vi "Open file simple via system exec.vi"(0 "file path":path) -> (4 "command line":string, 15 "error out":errorcluster)   [LabVIEW 2013]
doc: "Opens the file via a simple System exec call.\nFails if hte file is already used by another process. Example: Access Database file is use by Prosis. Then this command fails."
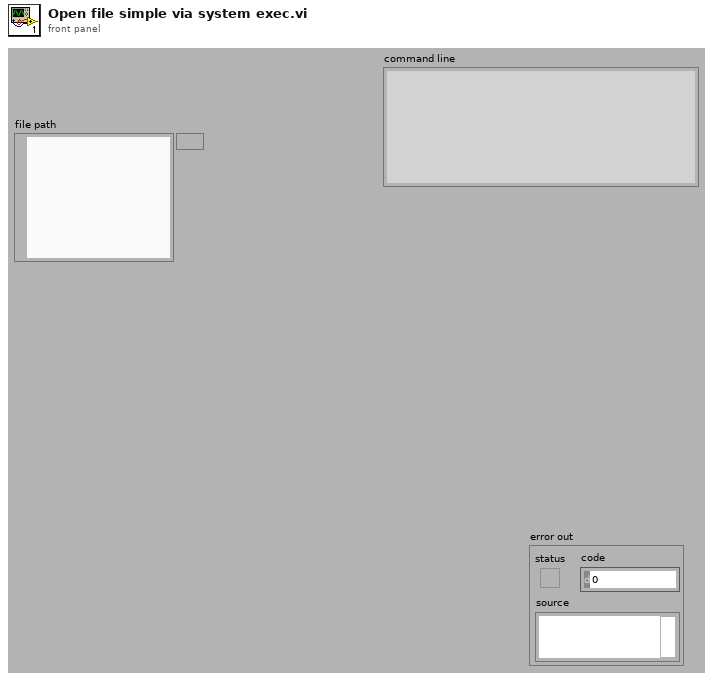
[diagram p1: front panel]
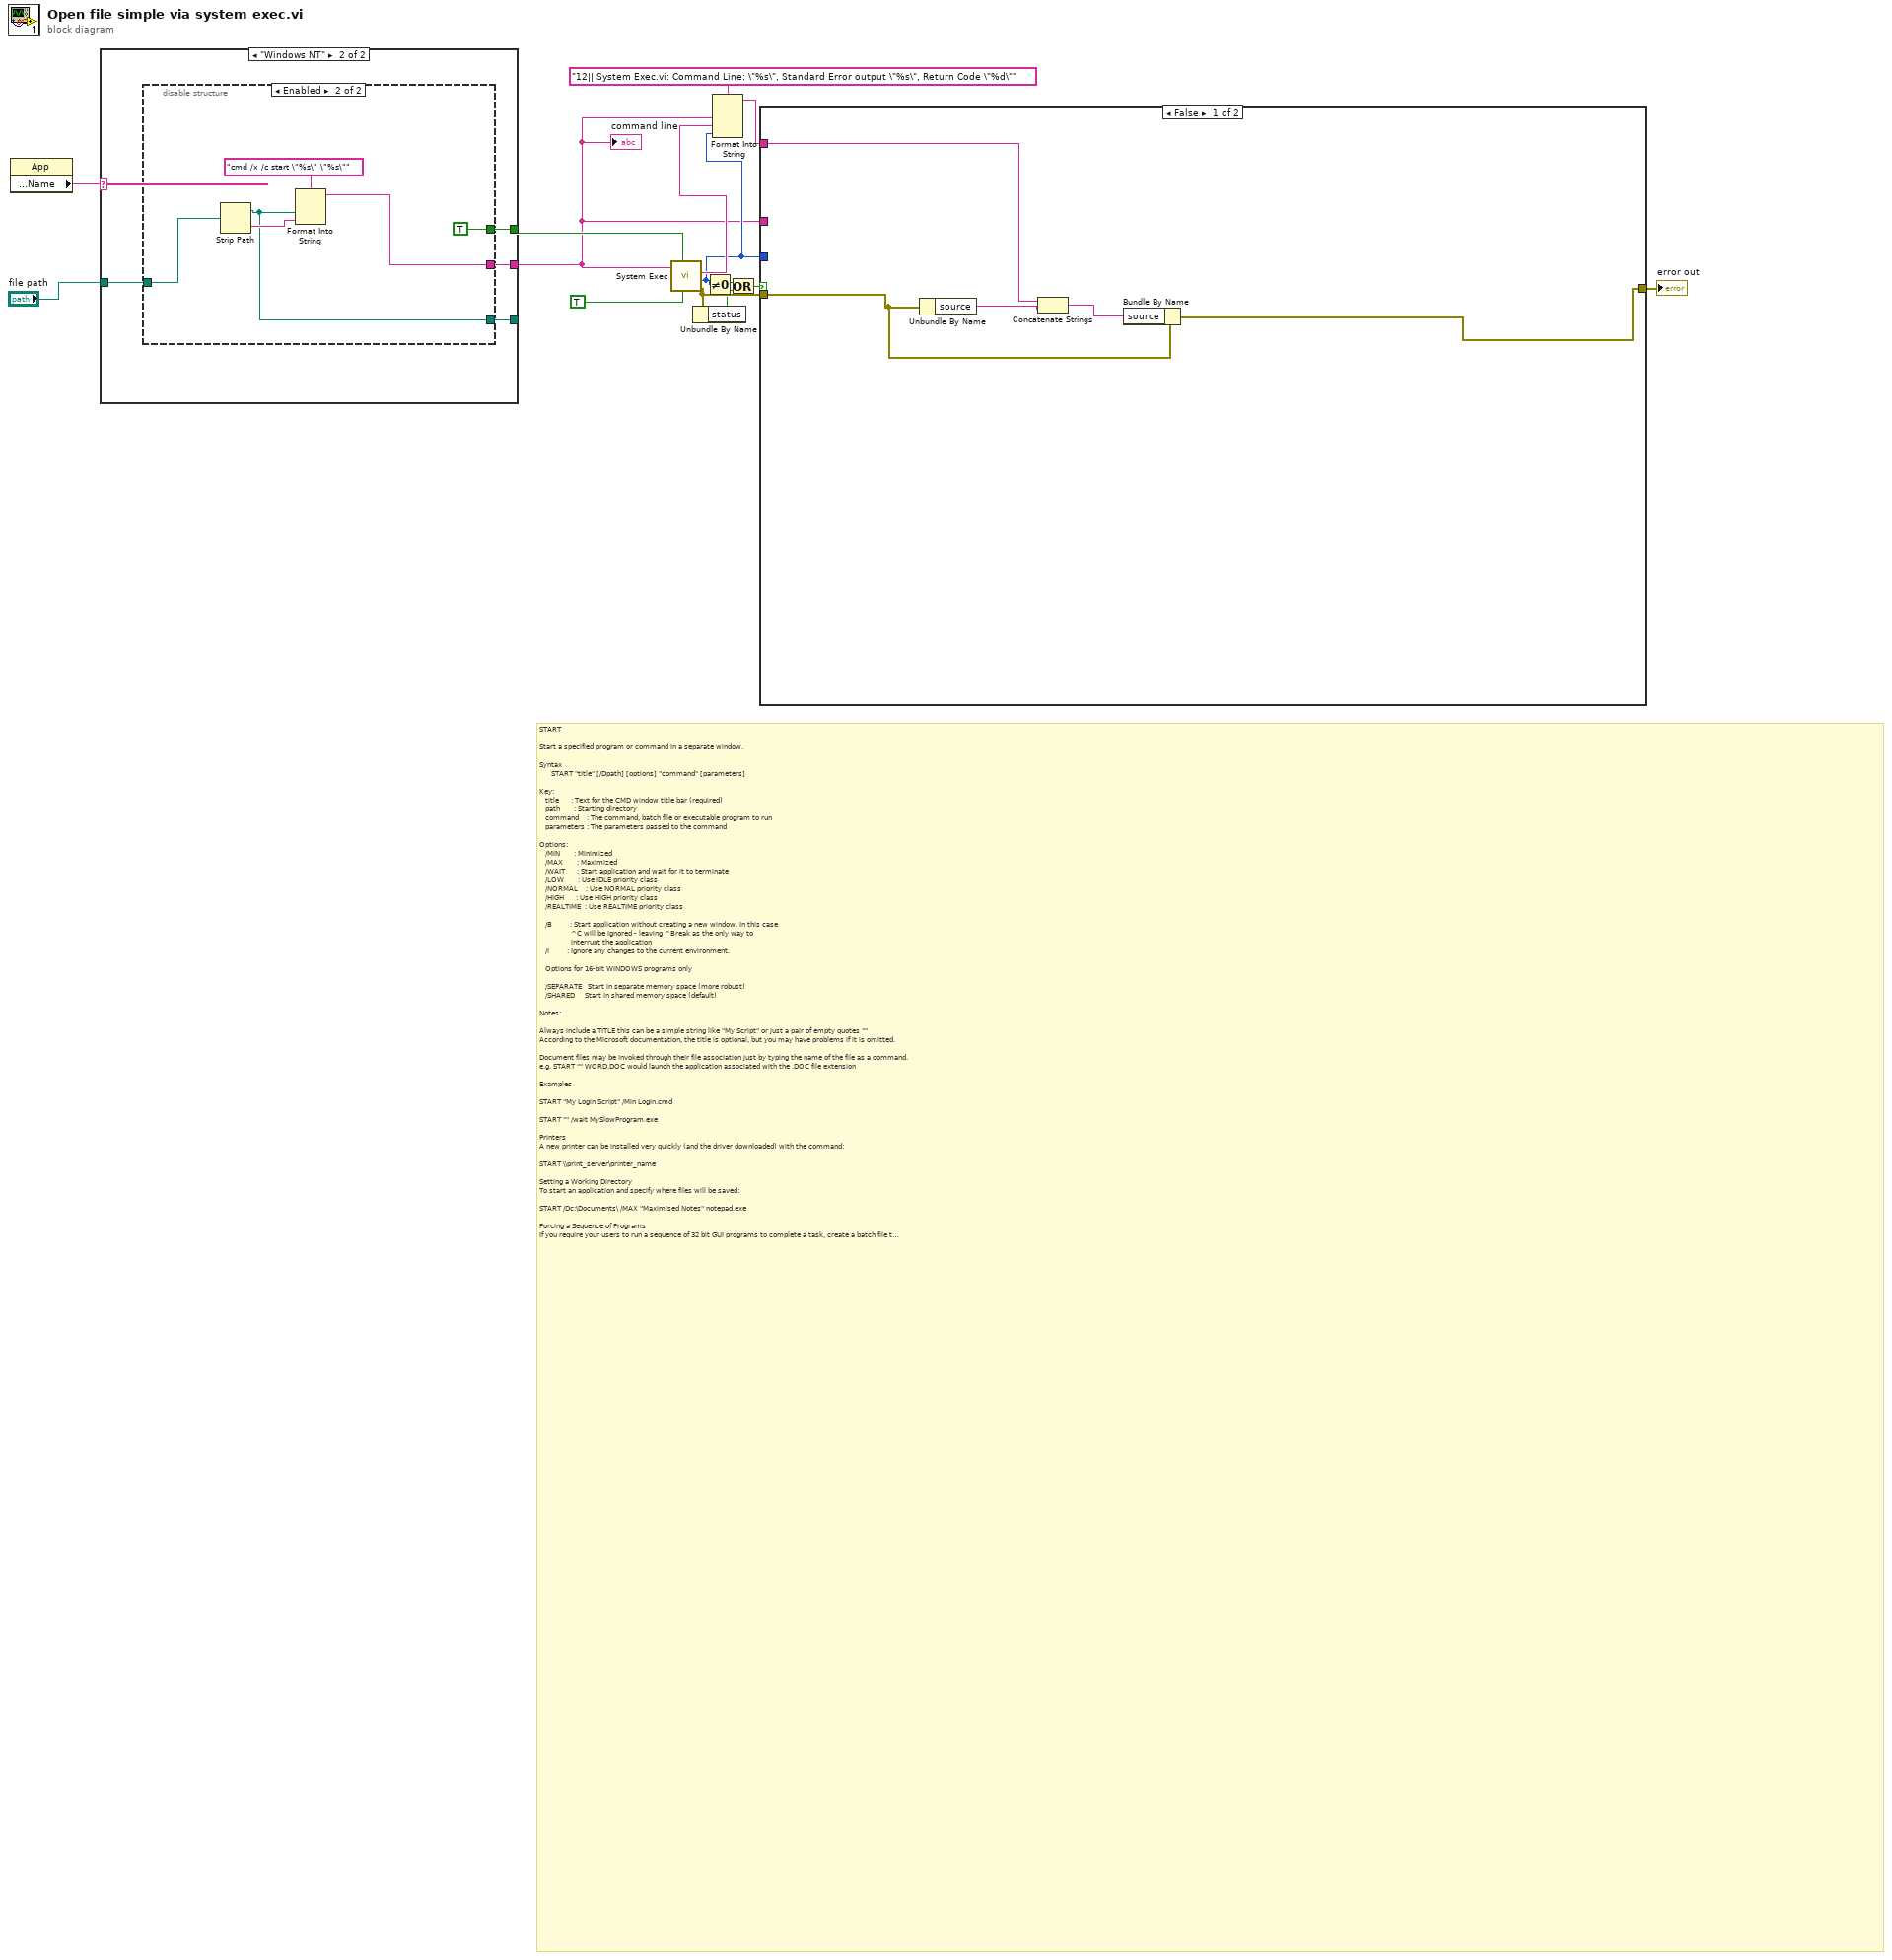
[diagram p0: block diagram]
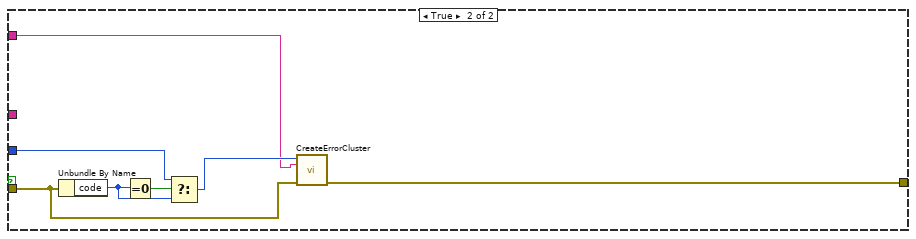
[diagram p2: hidden frame]
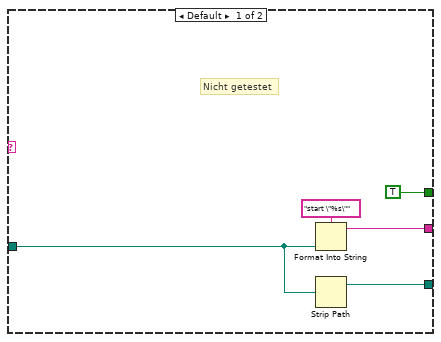
[diagram p3: hidden frame]
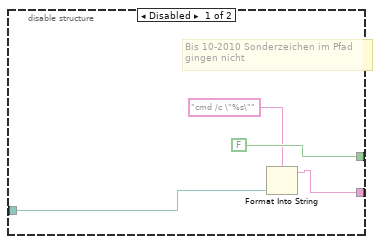
[diagram p4: hidden frame]
diagram:
  # "START\n\nStart a specified program or command in a separate window.\n\nSyntax\n      START \"title\" [/Dpath] [options] \"command\" [parameters]\n\nKey:\n   title      : Text for the CMD window title bar (required)\n   path       : Starting directory\n   command    : The command, batch file or executable program to run\n   parameters : The parameters passed to the command\n\nOptions:\n   /MIN       : Minimized\n   /MAX       : Maximized\n   /WAIT      : Start application and wait for it to terminate\n   /LOW       : Use IDLE priority class\n   /NORMAL    : Use NORMAL priority class\n   /HIGH      : Use HIGH priority class\n   /REALTIME  : Use REALTIME priority class\n\n   /B         : Start application without creating a new window. In this case\n                ^C will be ignored - leaving ^Break as the only way to \n                interrupt the application\n   /I         : Ignore any changes to the current environment.\n\n   Options for 16-bit WINDOWS programs only\n\n   /SEPARATE   Start in separate memory space (more robust)\n   /SHARED     Start in shared memory space (default)\n\nNotes:\n\nAlways include a TITLE this can be a simple string like \"My Script\" or just a pair of empty quotes \"\"\nAccording to the Microsoft documentation, the title is optional, but you may have problems if it is omitted.\n\nDocument files may be invoked through their file association just by typing the name of the file as a command.\ne.g. START \"\" WORD.DOC would launch the application associated with the .DOC file extension\n\nExamples\n\nSTART \"My Login Script\" /Min Login.cmd\n\nSTART \"\" /wait MySlowProgram.exe\n\nPrinters\nA new printer can be installed very quickly (and the driver downloaded) with the command:\n\nSTART \\\\print_server\\printer_name\n\nSetting a Working Directory\nTo start an application and specify where files will be saved:\n\nSTART /Dc:\\Documents\\ /MAX \"Maximised Notes\" notepad.exe\n\nForcing a Sequence of Programs\nIf you require your users to run a sequence of 32 bit GUI programs to complete a task, create a batch file that uses the start command:\n\n@echo off\nstart /wait /b First.exe\nstart /wait /b Second.exe\nstart /wait /b Third.exe\n\nCreate a shortcut to this batch file and place it on the Start menu or desktop. Set it to run minimized.\nWhen the user double-clicks the shortcut, <First.exe> runs.\nWhen <First.exe> terminates, <Second.exe> runs\nWhen <Second.exe> terminates, <Third.exe> runs\n\nAn alternative method is to run a .BAT batch file under command.com (16 bit)\n\nIf Command Extensions are disabled, the START command will no longer recognise file Associations, and will not automatically evaluate the COMSPEC variable when starting a second CMD session.\n\nMissing file extensions\nWhen executing a command line whose first token does NOT contain an extension, then CMD.EXE uses the value of the PATHEXT environment variable to determine which extensions to look for and in what order. The default value for the PATHEXT variable is:\n\n.COM;.EXE;.BAT;.CMD\n\nNotice the syntax is the same as the PATH variable, with semicolons separating the different elements.\n\nWhen executing a command, if there is no match on any extension, then Windows will look to see if the name, without any extension, matches a directory name and if it does, the START command will launch Explorer on that path.\n\n\"Do not run; scorn running with thy heels\" - Shakespeare, The Merchant of Venice"
  n1 = property class="App"() -> ("Operating System:Name"=w8:string)  [unwired: 2 in, 2 out]
  n2 = case shown="\"Windows NT\"" w8 {
    tunnel: [TRUE ("wait until completion? (T)") w23] -> w9
    tunnel: "file path" -> [w16 w21]
    tunnel: [w17 w22] -> w1
    tunnel: [w15 w20] -> _
    frame Default {
      # "Nicht getestet"
      n3 = Format Into String(format string="start \"%s\"" ("Input 1"), w16) -> (resulting string=w17:string)  [unwired: 2 in, 1 out]
      n4 = Strip Path(path=w16) -> (stripped path=w15:path)  [unwired: 1 out]
    }
    frame "Windows NT" {
      n5 = disable-structure shown="Enabled" {
        disable-tunnel: [FALSE ("wait until completion? (T)") TRUE ("wait until completion? (T)")] -> w23
        disable-tunnel: [w26 w31] -> w22
        disable-tunnel: w21 -> [w24 w33]
        disable-tunnel: [_ w28] -> w20
        frame Disabled {
          # "Bis 10-2010 Sonderzeichen im Pfad \ngingen nicht"
          n6 = Format Into String(format string="cmd /c \"%s\"" ("Input 1"), w24) -> (resulting string=w26:string)  [unwired: 2 in, 1 out]
        }
        frame Enabled {
          n7 = Strip Path(path=w33) -> (stripped path=w28:path, name=w32:string)
          n8 = Format Into String(format string="cmd /x /c start \"%s\" \"%s\"" ("string"), w28, w32) -> (resulting string=w31:string)  [unwired: 2 in, 1 out]
        }
      }
    }
  }
  "command line" <- w1
  n9 = call <vilib>:"System Exec.vi"("run minimized? (F)"=TRUE, "wait until completion? (T)"=w9, "command line"=w1) -> ("error out"=w14:errorcluster, "return code"=w4:i32, "standard error"=w6:string)  [unwired: 5 in, 1 out]
  n10 = Unbundle By Name(w14) -> ("status"=w12:bool)
  n11 = Not Equal To 0?(x=w4) -> (x != 0?=w11:bool)
  n12 = Format Into String(format string="12|| System Exec.vi: Command Line: \"%s\", Standard Error output \"%s\", Return Code \"%d\"", w1, w6, w4) -> (resulting string=w3:string)  [unwired: 2 in, 1 out]
  n13 = Or(x=w11, y=w12) -> (x .or. y?=w13:bool)
  n14 = case shown="False" w13 {
    tunnel: [w35 w45] -> w10
    tunnel: w1 -> [_ _]
    tunnel: w4 -> [_ w44]
    tunnel: w14 -> [w38 w43]
    tunnel: w3 -> [w34 w39]
    frame False {
      n15 = Unbundle By Name(w38) -> ("source"=w37:string)
      n16 = Concatenate Strings(w34, w37) -> (w36:string)
      n17 = Bundle By Name(cluster=w38, "source"=w36) -> (w35:errorcluster)
    }
    frame True {
      n18 = Unbundle By Name(w43) -> ("code"=w41:i32)
      n19 = Equal To 0?(x=w41) -> (x = 0?=w42:bool)
      n20 = Select(t=w44, s=w42, f=w41) -> (s? t:f=w40:i32)
      n21 = call "CreateErrorCluster.vi"("Error Code"=w40, "Additional description"=w39, "error in"=w43) -> ("error out"=w45:errorcluster)  [unwired: 12 in]
    }
  }
  "error out" <- w10
